vi "App.vi"() -> ()   [LabVIEW 2015]
uses:
  <vilib>/DAQmx/read.llb/DAQmx Read (Analog DBL 1Chan 1Samp).vi
  <vilib>/DAQmx/read.llb/DAQmx Read (Analog Wfm 1Chan NSamp).vi
  <vilib>/DAQmx/miscellaneous.llb/DAQmx Fill In Error Info.vi
panel:
  in  "task out":refnum<k21>
  out "Button 2":u16
  out "Waveform Chart 2":waveform(dbl)
  out "Button":u16
  in  "Tab Control":T1(tab)
  in  "Zoom":bool
  in  "Vol (AI3/AI7)":bool
  out "min value":dbl format="%#.2f"
  out "max value":dbl format="%#.2f"
  out "Delta(ms)":dbl format="%#_5f"
  in  "Zero":bool
  out "Average":dbl format="%#_4g"
  in  "mA/uA":bool
  out "Waveform Graph":waveform(dbl)(graph)
  in  "uA/mA":bool=TRUE
  out "Waveform Graph 2":waveform(dbl)(graph)
  out "Average (uA)":dbl
  in  "PAUSE":bool
  out "Vbat":dbl
  out "Waveform Chart":dbl(graph)
  in  "Number of samples uC Board":i32=10000
  in  "USB DAQ":tag="Dev1"
  in  "Stream":bool
  out "Waveform Chart 3":dbl(graph)
  in  "file List":i32(listbox)
  out "2D Picture":picture
  # "FW Validation - Current Tracking V1.0"
  # "For uC Board: 20kS/s"
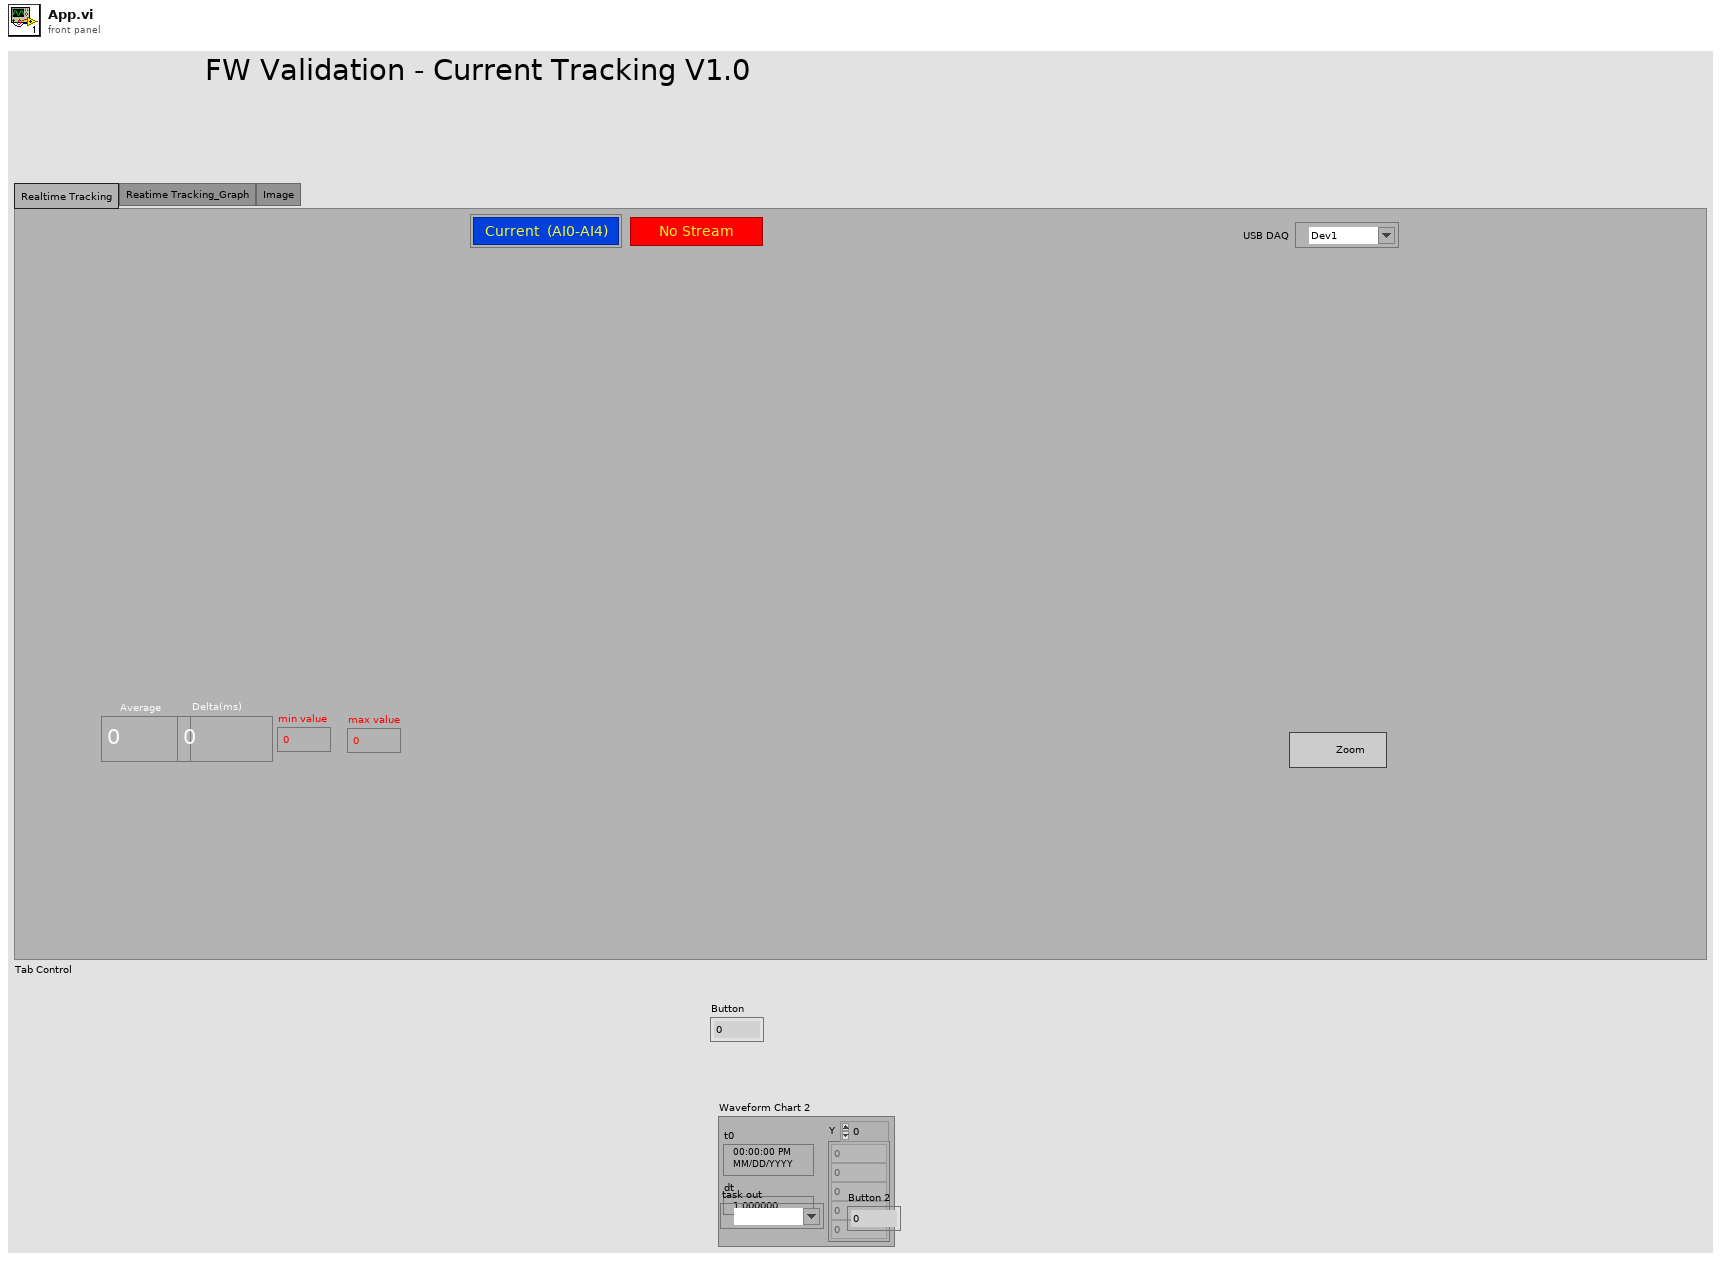
[diagram p1: front panel]
types:
  T1 = enum32{"Realtime Tracking", "Reatime Tracking_Graph", "Image"}
  T2 = typedef "imagedata.ctl" = cluster{"image type":i32, "image depth":i32, "image":u8[], "mask":u8[], "colors":u32[], "Rectangle":cluster{"left":i16, "top":i16, "right":i16, "bottom":i16}}
  T3 = typedef "LVCursorListTypeDef.ctl" = cluster{"Name":string, "Color":u32, "Style":u8, "Point Style":u8, "Name Visible":bool, "Allow Drag":bool, "Cursor Mode":u32, "Plot":i32, "Index":i32, "Position":cluster{"X":dbl, "Y":dbl}, "X Scale":u32, "Y Scale":u32, "Watch Plots":i32[], "Watch All Plots":bool, "Plot Area":i32, "Label Offset":cluster{"X":dbl, "Y":dbl}}[]
  T4 = cluster{"Name":string, "Color":u32, "Style":u8, "Point Style":u8, "Name Visible":bool, "Allow Drag":bool, "Cursor Mode":u32, "Plot":i32, "Index":i32, "Position":cluster{"X":dbl, "Y":dbl}, "X Scale":u32, "Y Scale":u32, "Watch Plots":i32[], "Watch All Plots":bool, "Plot Area":i32, "Label Offset":cluster{"X":dbl, "Y":dbl}}
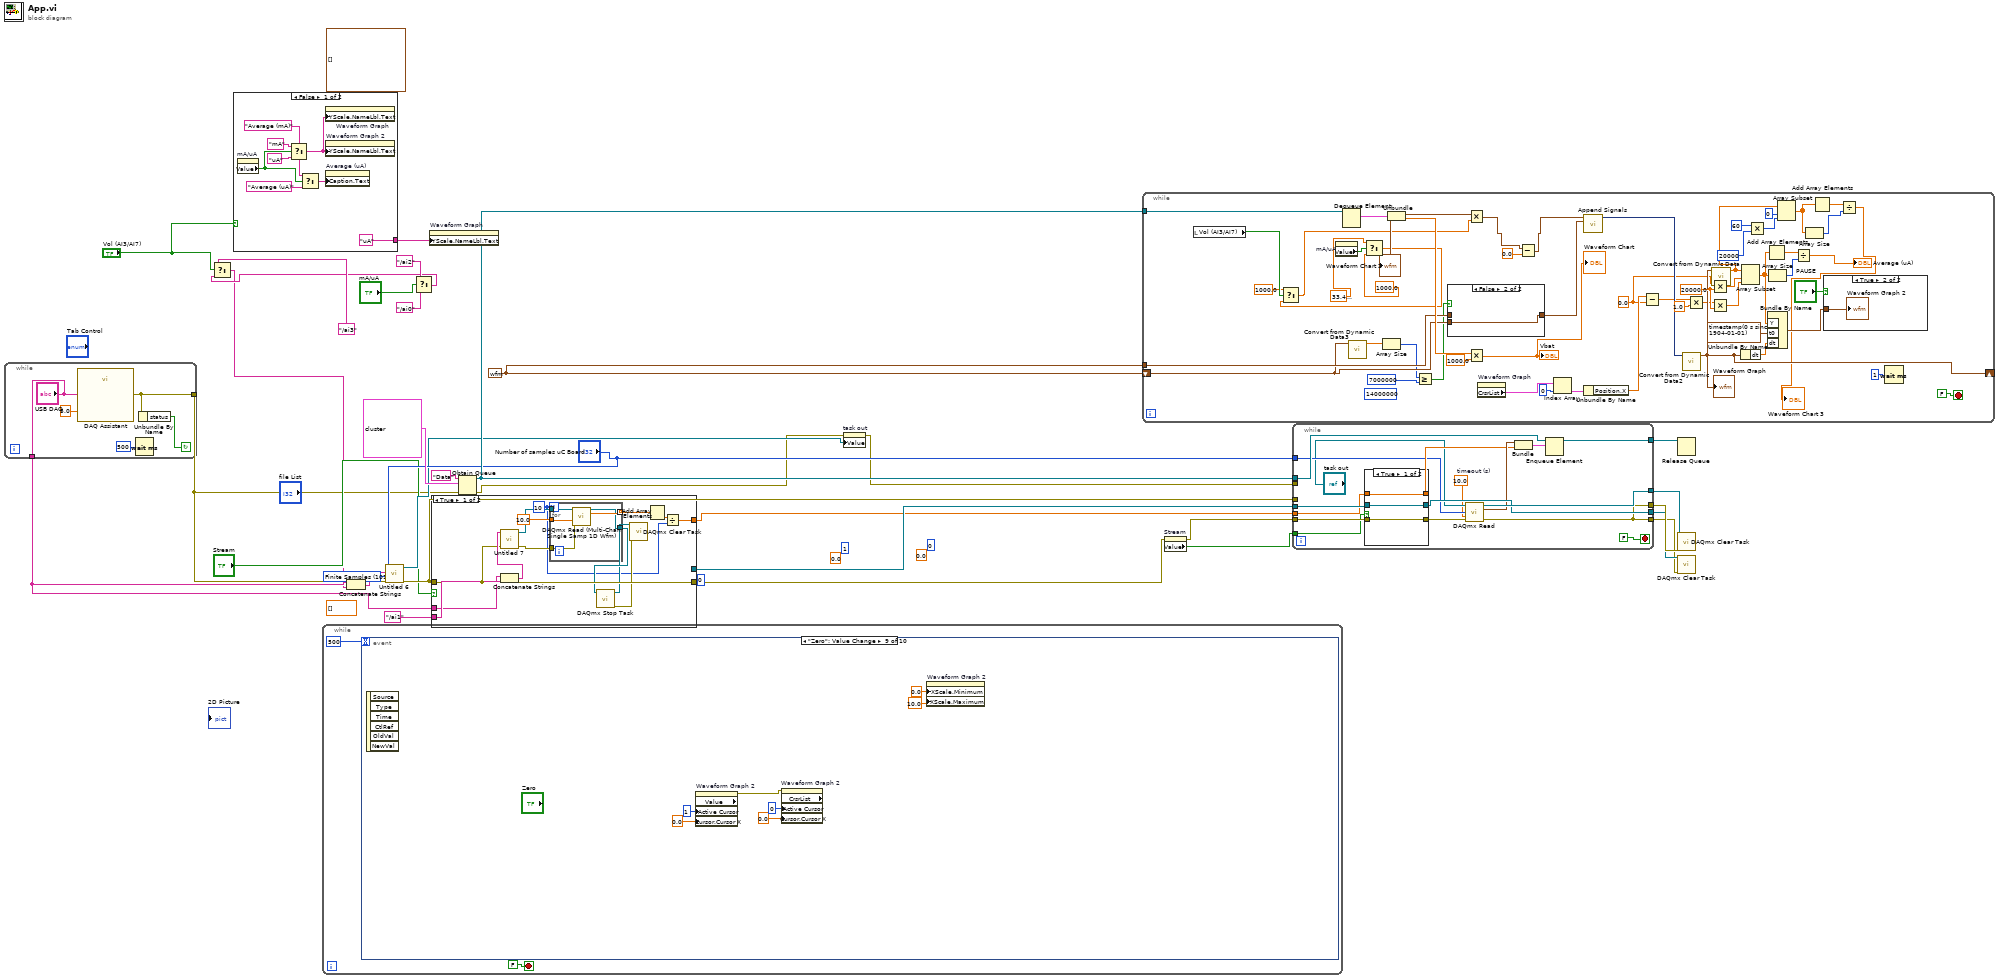
[diagram p0: block diagram]
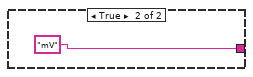
[diagram p2: hidden frame]
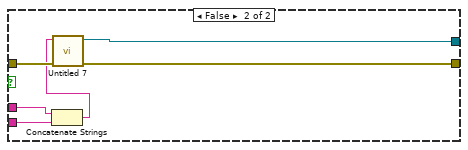
[diagram p3: hidden frame]
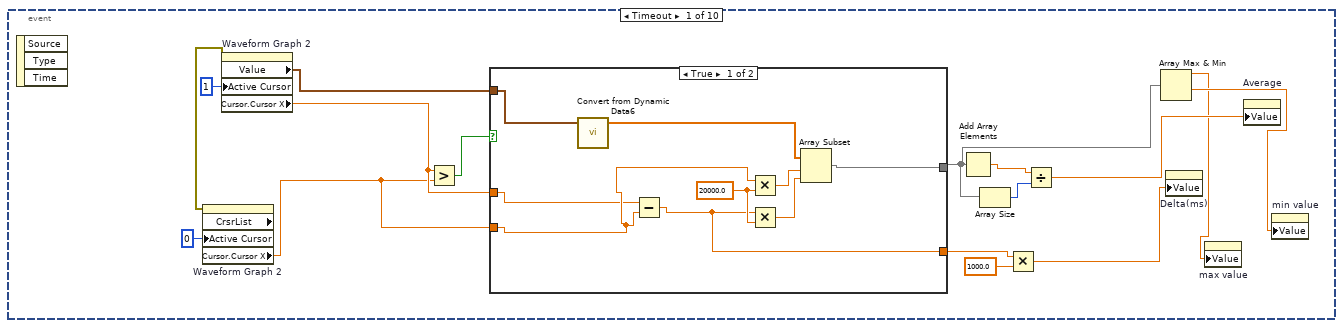
[diagram p4: hidden frame]
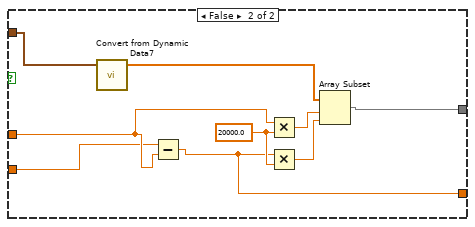
[diagram p5: hidden frame]
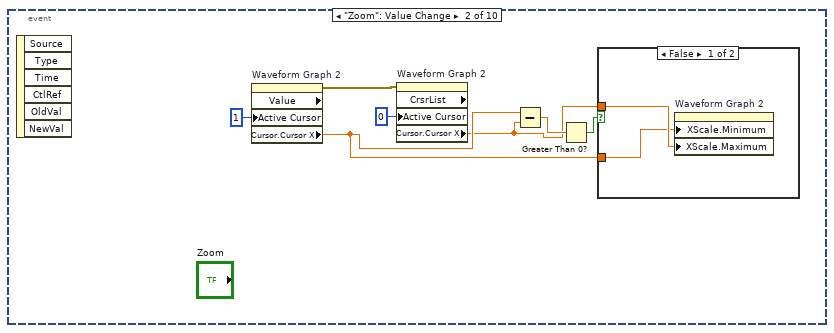
[diagram p6: hidden frame]
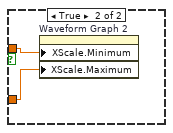
[diagram p7: hidden frame]
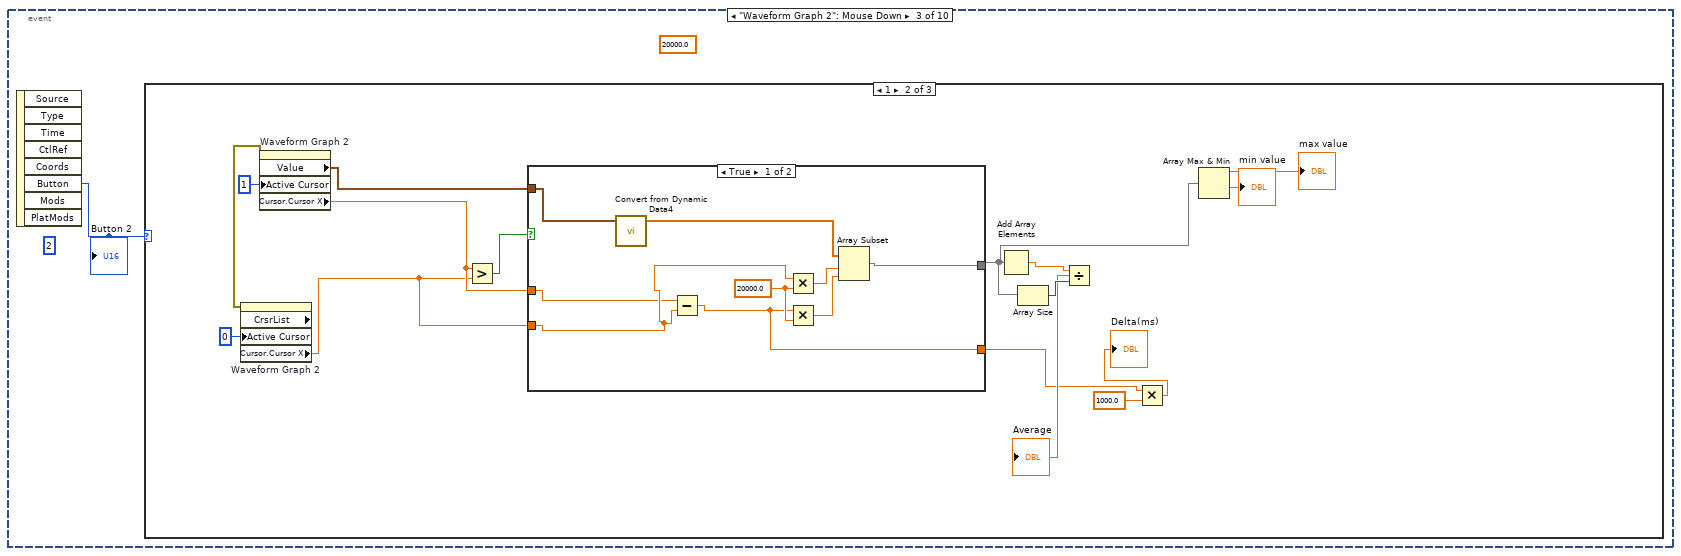
[diagram p8: hidden frame]
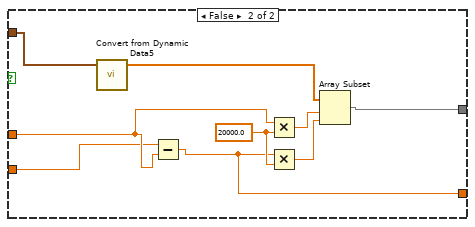
[diagram p10: hidden frame]
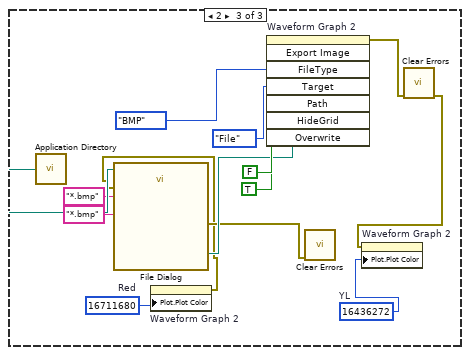
[diagram p11: hidden frame]
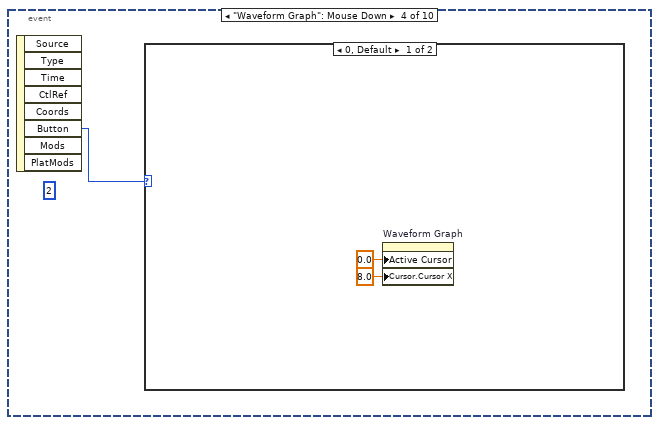
[diagram p12: hidden frame]
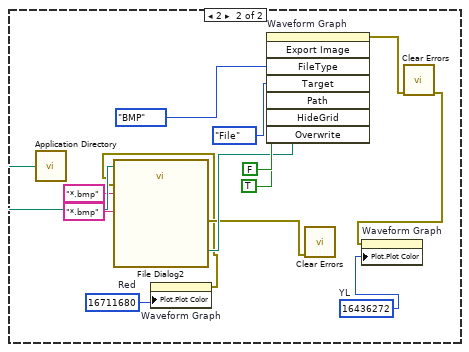
[diagram p13: hidden frame]
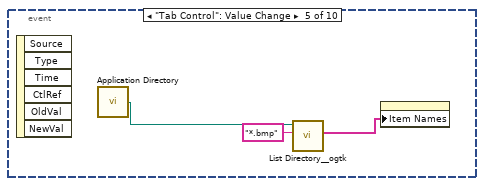
[diagram p14: hidden frame]
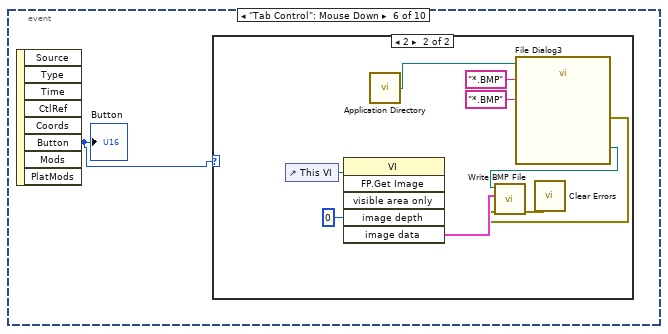
[diagram p15: hidden frame]
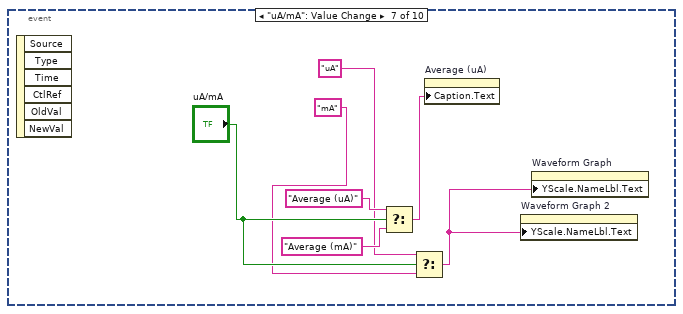
[diagram p17: hidden frame]
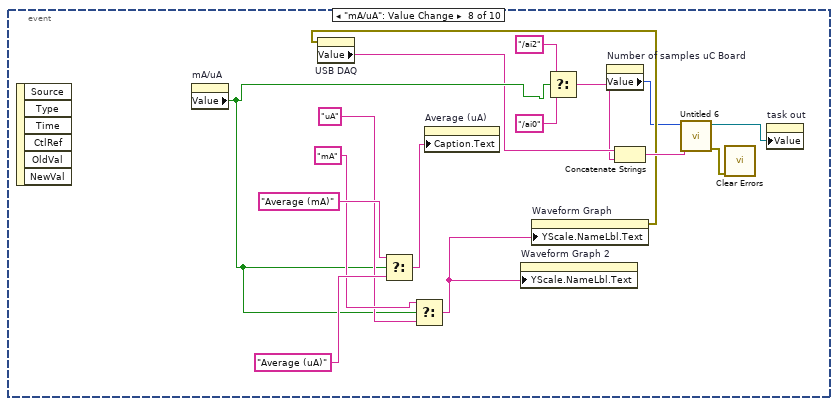
[diagram p18: hidden frame]
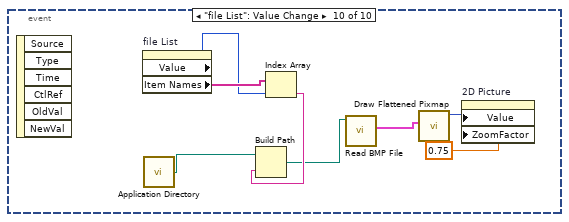
[diagram p19: hidden frame]
diagram:
  (unwired) 0.0 ("Cursor.Cursor Position:Cursor X")
  (unwired) 0.0 ("Cursor.Cursor Position:Cursor X")
  (unwired) u32 0 ("Active Cursor")
  (unwired) u32 1 ("Active Cursor")
  w13 = 10178 items=["Finite Samples"=10178, "Continuous Samples"=10123, "Hardware Timed Single Point"=12522] ("sample mode")
  (unwired) u32 0 ("Active Cursor")
  w23 = waveform(dbl) {"t0"=timestamp(0 s since 1904-01-01), "dt"=0.0, "Y"=[]} ("data")
  (unwired) waveform(dbl)[] [] ("History Data")
  (unwired) dbl[] [] ("Array")
  n1 = while {
    tunnel: [w36] -> w6
    tunnel: ["USB DAQ"] -> w20
    stop <- w35 continue-if-true
    n2 = call "DAQ Assistant"("data"=5.0, "device name"="USB DAQ") -> ("error out"=w36:errorcluster)  [unwired: 16 in, 1 out]
    n3 = Wait (ms)(milliseconds to wait=u32 500) -> ()  [unwired: 1 out]
    n4 = Unbundle By Name(w36) -> ("status"=w35:bool)
  }
  n5 = case shown="False" "Vol (AI3/AI7)" {
    tunnel: ["uA" ("Y Scale.Name Label.Text") "mV" ("Y Scale.Name Label.Text")] -> w1
    frame False {
      n6 = property on="mA/uA" class="Bool (strict)"() -> ("Value"=w43:bool)  [unwired: 2 in, 2 out]
      n7 = Select(t="mA" ("Caption.Text"), s=w43, f="uA" ("Caption.Text")) -> (s? t:f=w44:string)
      n8 = Select(t="Average (mA)" ("Caption.Text"), s=w43, f="Average (uA)" ("Caption.Text")) -> (s? t:f=w45:string)
      n9 = property on="Waveform Graph" class="WFGraph (strict)"("YScale.NameLbl.Text"=w44) -> ()  [unwired: 2 in, 2 out]
      n10 = property on="Waveform Graph 2" class="WFGraph (strict)"("YScale.NameLbl.Text"=w44) -> ()  [unwired: 2 in, 2 out]
      n11 = property on="Average (uA)" class="DigNum (strict)"("Caption.Text"=w45) -> ()  [unwired: 2 in, 2 out]
    }
    frame True {
    }
  }
  n12 = while {
    stop <- FALSE stop-if-true
    n13 = event shown="[8] \"Zero\": Value Change" {
      selector: _ -> [_ _ _ _ _ _ _ _ _ _]
      dyn-events: _ -> [_ _ _ _ _ _ _ _ _ _]
      timeout: 500 -> [_ _ _ _ _ _ _ _ _ _]
      event Timeout {
        n14 = event-data() -> ()  [unwired: 1 in, 3 out]
        n15 = property on="Waveform Graph 2" class="WFGraph (strict)"("Active Cursor"=u32 1) -> (error out=w60:errorcluster, "Value"=w56:waveform(dbl), "Cursor.Cursor X"=w62:dbl)  [unwired: 2 in, 1 out]
        n16 = property on="Waveform Graph 2" class="WFGraph (strict)" props=["CrsrList", "Active Cursor", "Cursor", "Cursor X"](error in=w60, "Active Cursor"=u32 0) -> ("Cursor.Cursor X"=w61:dbl)  [unwired: 1 in, 3 out]
        n17 = Greater?(x=w62, y=w61) -> (0:w63:bool)
        n18 = case shown="True" w63 {
          tunnel: w56 -> [w74 w83]
          tunnel: w62 -> [w67 w77]
          tunnel: w61 -> [w68 w76]
          tunnel: [w69 w78] -> w57
          tunnel: [w66 w75] -> w52
          frame True {
            w72 = 20000.0 ("y")
            n19 = call "Convert from Dynamic Data6"("Dynamic Data Type"=w74) -> ("Array"=w70:dbl[])  [unwired: 3 in]
            n20 = Subtract(x=w67, y=w68) -> (x-y=w66:dbl)
            n21 = Multiply(x=w68, y=w72) -> (x*y=w73:dbl)
            n22 = Multiply(x=w66, y=w72) -> (x*y=w71:dbl)
            n23 = Array Subset(array=w70, index=w73, length=w71) -> (w69:dbl[])
          }
          frame False {
            w81 = 20000.0 ("y")
            n24 = call "Convert from Dynamic Data7"("Dynamic Data Type"=w83) -> ("Array"=w79:dbl[])  [unwired: 3 in]
            n25 = Subtract(x=w76, y=w77) -> (x-y=w75:dbl)
            n26 = Multiply(x=w77, y=w81) -> (x*y=w82:dbl)
            n27 = Multiply(x=w75, y=w81) -> (x*y=w80:dbl)
            n28 = Array Subset(array=w79, index=w82, length=w80) -> (w78:dbl[])
          }
        }
        n29 = Add Array Elements(numeric array=w57) -> (sum=w59:dbl)
        n30 = Array Size(array=w57) -> (size(s)=w58:i32)
        n31 = Multiply(x=w52, y=1000.0) -> (x*y=w51:dbl)
        n32 = Divide(x=w59, y=w58) -> (x/y=w55:dbl)
        n33 = Array Max & Min(array=w57) -> (max value=w53:dbl, min value=w54:dbl)  [unwired: 2 out]
        n34 = property on="Delta(ms)" class="DigNum (strict)"("Value"=w51) -> ()  [unwired: 2 in, 2 out]
        n35 = property on="max value" class="DigNum (strict)"("Value"=w53) -> ()  [unwired: 2 in, 2 out]
        n36 = property on="Average" class="DigNum (strict)"("Value"=w55) -> ()  [unwired: 2 in, 2 out]
        n37 = property on="min value" class="DigNum (strict)"("Value"=w54) -> ()  [unwired: 2 in, 2 out]
      }
      event "Zoom": Value Change {
        n38 = event-data() -> ()  [unwired: 1 in, 6 out]
        n39 = property on="Waveform Graph 2" class="WFGraph (strict)" props=["Value", "Active Cursor", "Cursor", "Cursor X"]("Active Cursor"=u32 1) -> (error out=w88:errorcluster, "Cursor.Cursor X"=w86:dbl)  [unwired: 2 in, 2 out]
        n40 = property on="Waveform Graph 2" class="WFGraph (strict)" props=["CrsrList", "Active Cursor", "Cursor", "Cursor X"](error in=w88, "Active Cursor"=u32 0) -> ("Cursor.Cursor X"=w85:dbl)  [unwired: 1 in, 3 out]
        n41 = Subtract(x=w86, y=w85) -> (x-y=w87:dbl)
        n42 = Greater Than 0?(x=w87) -> (x > 0?=w84:bool)
        n43 = case shown="False" w84 {
          tunnel: w86 -> [w91 w94]
          tunnel: w85 -> [w92 w93]
          frame False {
            n44 = property on="Waveform Graph 2" class="WFGraph (strict)"("XScale.Minimum"=w91, "XScale.Maximum"=w92) -> ()  [unwired: 2 in, 2 out]
          }
          frame True {
            n45 = property on="Waveform Graph 2" class="WFGraph (strict)"("XScale.Minimum"=w93, "XScale.Maximum"=w94) -> ()  [unwired: 2 in, 2 out]
          }
        }
      }
      event "Waveform Graph 2": Mouse Down {
        (unwired) 20000.0 ("y")
        (unwired) u16 2 ("Button")
        n46 = event-data() -> ("Button"=w95:u16)  [unwired: 1 in, 7 out]
        "Button 2" <- w95
        n47 = case shown="1" w95 {
          frame 0, Default {
          }
          frame 1 {
            n48 = property on="Waveform Graph 2" class="WFGraph (strict)"("Active Cursor"=u32 1) -> (error out=w106:errorcluster, "Value"=w99:waveform(dbl), "Cursor.Cursor X"=w108:dbl)  [unwired: 2 in, 1 out]
            n49 = property on="Waveform Graph 2" class="WFGraph (strict)" props=["CrsrList", "Active Cursor", "Cursor", "Cursor X"](error in=w106, "Active Cursor"=u32 0) -> ("Cursor.Cursor X"=w107:dbl)  [unwired: 1 in, 3 out]
            n50 = Greater?(x=w108, y=w107) -> (0:w109:bool)
            n51 = case shown="True" w109 {
              tunnel: w99 -> [w120 w129]
              tunnel: w108 -> [w113 w123]
              tunnel: w107 -> [w114 w122]
              tunnel: [w115 w124] -> w102
              tunnel: [w112 w121] -> w96
              frame True {
                w118 = 20000.0 ("y")
                n52 = call "Convert from Dynamic Data4"("Dynamic Data Type"=w120) -> ("Array"=w116:dbl[])  [unwired: 3 in]
                n53 = Subtract(x=w113, y=w114) -> (x-y=w112:dbl)
                n54 = Multiply(x=w114, y=w118) -> (x*y=w119:dbl)
                n55 = Multiply(x=w112, y=w118) -> (x*y=w117:dbl)
                n56 = Array Subset(array=w116, index=w119, length=w117) -> (w115:dbl[])
              }
              frame False {
                w127 = 20000.0 ("y")
                n57 = call "Convert from Dynamic Data5"("Dynamic Data Type"=w129) -> ("Array"=w125:dbl[])  [unwired: 3 in]
                n58 = Subtract(x=w122, y=w123) -> (x-y=w121:dbl)
                n59 = Multiply(x=w123, y=w127) -> (x*y=w128:dbl)
                n60 = Multiply(x=w121, y=w127) -> (x*y=w126:dbl)
                n61 = Array Subset(array=w125, index=w128, length=w126) -> (w124:dbl[])
              }
            }
            n62 = Add Array Elements(numeric array=w102) -> (sum=w105:dbl)
            n63 = Array Size(array=w102) -> (size(s)=w104:i32)
            n64 = Divide(x=w105, y=w104) -> (x/y=→"Average":dbl)
            n65 = Multiply(x=w96, y=1000.0) -> (x*y=→"Delta(ms)":dbl)
            n66 = Array Max & Min(array=w102) -> (max value=→"max value":dbl, min value=→"min value":dbl)  [unwired: 2 out]
          }
          frame 2 {
            w130 = u32 16436272  # YL
            w132 = u32 16711680  # Red
            n67 = call <vilib>:"Application Directory.vi"() -> ("Application Directory"=w139:path)
            n68 = property on="Waveform Graph 2" class="WFGraph (strict)"("Plot.Plot Color"=w132) -> (error out=w133:errorcluster)  [unwired: 2 in, 1 out]
            n69 = call "File Dialog"("start path"=w139, "error in"=w133, "pattern (all files)"="*.bmp", "pattern label"="*.bmp") -> ("selected path"=w136:path, "error out"=w135:errorcluster)  [unwired: 8 in, 2 out]
            n70 = invoke on="Waveform Graph 2" class="WFGraph (strict)" method="Export Image"("FileType"=enum32{"BMP", "EPS", "EMF", "PICT"}."BMP" ("File Type"), "Target"=enum32{"File", "Clipboard"}."File", "Path"=w136, "HideGrid"=FALSE ("Hide Grid"), "Overwrite"=TRUE ("Always Overwrite")) -> (error out=w134:errorcluster)  [unwired: 3 in, 7 out]
            n71 = call <vilib>:"Clear Errors.vi"("error in (no error)"=w135) -> ()  [unwired: 5 in, 2 out]
            n72 = call <vilib>:"Clear Errors.vi"("error in (no error)"=w134) -> ("error out"=w131:errorcluster)  [unwired: 5 in, 1 out]
            n73 = property on="Waveform Graph 2" class="WFGraph (strict)"(error in=w131, "Plot.Plot Color"=w130) -> ()  [unwired: 1 in, 2 out]
          }
        }
      }
      event "Waveform Graph": Mouse Down {
        (unwired) u16 2 ("Button")
        n74 = event-data() -> ("Button"=w144:u16)  [unwired: 1 in, 7 out]
        n75 = case shown="0, Default" w144 {
          frame 0, Default {
            n76 = property on="Waveform Graph" class="WFGraph (strict)"("Active Cursor"=0.0 ("Cursor.Cursor Position:Cursor X"), "Cursor.Cursor X"=8.0 ("Cursor.Cursor Position:Cursor X")) -> ()  [unwired: 2 in, 2 out]
          }
          frame 2 {
            w147 = u32 16436272  # YL
            w149 = u32 16711680  # Red
            n77 = call <vilib>:"Application Directory.vi"() -> ("Application Directory"=w156:path)
            n78 = property on="Waveform Graph" class="WFGraph (strict)"("Plot.Plot Color"=w149) -> (error out=w150:errorcluster)  [unwired: 2 in, 1 out]
            n79 = call "File Dialog2"("start path"=w156, "error in"=w150, "pattern (all files)"="*.bmp", "pattern label"="*.bmp") -> ("selected path"=w153:path, "error out"=w152:errorcluster)  [unwired: 8 in, 2 out]
            n80 = invoke on="Waveform Graph" class="WFGraph (strict)" method="Export Image"("FileType"=enum32{"BMP", "EPS", "EMF", "PICT"}."BMP" ("File Type"), "Target"=enum32{"File", "Clipboard"}."File", "Path"=w153, "HideGrid"=FALSE ("Hide Grid"), "Overwrite"=TRUE ("Always Overwrite")) -> (error out=w151:errorcluster)  [unwired: 3 in, 7 out]
            n81 = call <vilib>:"Clear Errors.vi"("error in (no error)"=w152) -> ()  [unwired: 5 in, 2 out]
            n82 = call <vilib>:"Clear Errors.vi"("error in (no error)"=w151) -> ("error out"=w148:errorcluster)  [unwired: 5 in, 1 out]
            n83 = property on="Waveform Graph" class="WFGraph (strict)"(error in=w148, "Plot.Plot Color"=w147) -> ()  [unwired: 1 in, 2 out]
          }
        }
      }
      event "Tab Control": Value Change {
        n84 = event-data() -> ()  [unwired: 1 in, 6 out]
        n85 = call <vilib>:"Application Directory.vi"() -> ("Application Directory"=w163:path)
        n86 = call <userlib>:"List Directory__ogtk.vi"("pattern"="*.bmp", "directory path"=w163) -> ("file names"=w161:string[])  [unwired: 2 in, 3 out]
        n87 = property on="file List" class="LstBox (strict)"("Item Names"=w161) -> ()  [unwired: 2 in, 2 out]
      }
      event "Tab Control": Mouse Down {
        n88 = event-data() -> ("Button"=w164:u16)  [unwired: 1 in, 7 out]
        "Button" <- w164
        n89 = case shown="2" w164 {
          frame 0, Default {
          }
          frame 2 {
            n90 = control-ref of="This VI"() -> (w173:refnum<vi>)
            n91 = invoke class="VI" method="FP.Get Image"(reference=w173, "image depth"=0 ("Image Depth")) -> ("image data"=w171:T2)  [unwired: 4 in, 5 out]
            n92 = call <vilib>:"Application Directory.vi"() -> ("Application Directory"=w167:path)
            n93 = call "File Dialog3"("start path"=w167, "pattern (all files)"="*.BMP", "pattern label"="*.BMP") -> ("selected path"=w170:path, "error out"=w169:errorcluster)  [unwired: 9 in, 2 out]
            n94 = call <vilib>:"Write BMP File.vi"("error in (no error)"=w169, "image data"=w171, "path to BMP file"=w170) -> ("error out"=w165:errorcluster)  [unwired: 7 in, 1 out]
            n95 = call <vilib>:"Clear Errors.vi"("error in (no error)"=w165) -> ()  [unwired: 5 in, 2 out]
          }
        }
      }
      event "uA/mA": Value Change {
        n96 = event-data() -> ()  [unwired: 1 in, 6 out]
        n97 = Select(t="Average (uA)" ("Caption.Text"), s="uA/mA", f="Average (mA)" ("Caption.Text")) -> (s? t:f=w180:string)
        n98 = Select(t="uA" ("Caption.Text"), s="uA/mA", f="mA" ("Caption.Text")) -> (s? t:f=w174:string)
        n99 = property on="Average (uA)" class="DigNum (strict)"("Caption.Text"=w180) -> ()  [unwired: 2 in, 2 out]
        n100 = property on="Waveform Graph 2" class="WFGraph (strict)"("YScale.NameLbl.Text"=w174) -> ()  [unwired: 2 in, 2 out]
        n101 = property on="Waveform Graph" class="WFGraph (strict)"("YScale.NameLbl.Text"=w174) -> ()  [unwired: 2 in, 2 out]
      }
      event "mA/uA": Value Change {
        n102 = event-data() -> ()  [unwired: 1 in, 6 out]
        n103 = property on="mA/uA" class="Bool (strict)"() -> ("Value"=w188:bool)  [unwired: 2 in, 2 out]
        n104 = Select(t="Average (mA)" ("Caption.Text"), s=w188, f="Average (uA)" ("Caption.Text")) -> (s? t:f=w196:string)
        n105 = Select(t="mA" ("Caption.Text"), s=w188, f="uA" ("Caption.Text")) -> (s? t:f=w195:string)
        n106 = property on="Average (uA)" class="DigNum (strict)"("Caption.Text"=w196) -> ()  [unwired: 2 in, 2 out]
        n107 = property on="Waveform Graph 2" class="WFGraph (strict)"("YScale.NameLbl.Text"=w195) -> ()  [unwired: 2 in, 2 out]
        n108 = property on="Waveform Graph" class="WFGraph (strict)"("YScale.NameLbl.Text"=w195) -> (error out=w184:errorcluster)  [unwired: 2 in, 1 out]
        n109 = property on="USB DAQ" class="DAQmxName"(error in=w184) -> ("Value"=w186:string)  [unwired: 1 in, 2 out]
        n110 = Select(t="/ai2" ("string"), s=w188, f="/ai0" ("string")) -> (s? t:f=w185:string)
        n111 = property on="Number of samples uC Board" class="DigNum (strict)"() -> ("Value"=w183:i32)  [unwired: 2 in, 2 out]
        n112 = Concatenate Strings(w186, w185) -> (w187:string)
        n113 = call "Untitled 6.vi"("physical channel"=w187, "number of samples"=w183) -> ("error out"=w181:errorcluster, "task out"=w182:refnum<k21>)  [unwired: 8 in]
        n114 = call <vilib>:"Clear Errors.vi"("error in (no error)"=w181) -> ()  [unwired: 5 in, 2 out]
        n115 = property on="task out" class="DAQmxName (strict)"("Value"=w182) -> ()  [unwired: 2 in, 2 out]
      }
      event "Zero": Value Change {
        n116 = event-data() -> ()  [unwired: 1 in, 6 out]
        n117 = property on="Waveform Graph 2" class="WFGraph (strict)" props=["Value", "Active Cursor", "Cursor", "Cursor X"]("Active Cursor"=u32 1, "Cursor.Cursor X"=0.0 ("Cursor.Cursor Position:Cursor X")) -> (error out=w201:errorcluster)  [unwired: 2 in, 2 out]
        n118 = property on="Waveform Graph 2" class="WFGraph (strict)" props=["CrsrList", "Active Cursor", "Cursor", "Cursor X"](error in=w201, "Active Cursor"=u32 0, "Cursor.Cursor X"=0.0 ("Cursor.Cursor Position:Cursor X")) -> ()  [unwired: 1 in, 3 out]
        n119 = property on="Waveform Graph 2" class="WFGraph (strict)"("XScale.Minimum"=0.0 ("X Scale.Range:Minimum"), "XScale.Maximum"=10.0 ("X Scale.Range:Maximum")) -> ()  [unwired: 2 in, 2 out]
      }
      event "file List": Value Change {
        n120 = event-data() -> ()  [unwired: 1 in, 6 out]
        n121 = property on="file List" class="LstBox (strict)"() -> ("Value"=w210:i32, "Item Names"=w211:string[])  [unwired: 2 in, 2 out]
        n122 = call <vilib>:"Application Directory.vi"() -> ("Application Directory"=w207:path)
        n123 = Index Array(array=w211, index=w210) -> (element=w206:string)
        n124 = Build Path(base path=w207, name or relative path=w206) -> (appended path=w205:path)
        n125 = call <vilib>:"Read BMP File.vi"("path to BMP file"=w205) -> ("image data"=w209:T2)  [unwired: 8 in, 2 out]
        n126 = call <vilib>:"Draw Flattened Pixmap.vi"("image data"=w209) -> ("new picture"=w208:picture)  [unwired: 8 in]
        n127 = property on="2D Picture" class="Pict"("Value"=w208, "ZoomFactor"=sgl 0.75 ("Zoom Factor")) -> ()  [unwired: 2 in, 2 out]
      }
    }
  }
  n128 = Select(t="/ai2" ("string"), s="mA/uA", f="/ai0" ("string")) -> (s? t:f=w4:string)
  n129 = Select(t="/ai3" ("string"), s="Vol (AI3/AI7)", f=w4) -> (s? t:f=w3:string)
  n130 = Concatenate Strings(w20, w3) -> (w21:string)
  n131 = call "Untitled 6.vi"("error in"=w6, "sample mode"=w13, "physical channel"=w21, "number of samples"="Number of samples uC Board") -> ("error out"=w25:errorcluster, "task out"=w16:refnum<k21>)  [unwired: 6 in]
  n132 = property on="Waveform Graph" class="WFGraph (strict)"("YScale.NameLbl.Text"=w1) -> ()  [unwired: 2 in, 2 out]
  n133 = case shown="True" "Stream" {
    tunnel: [_ w236] -> w28
    tunnel: [w223 w235] -> w10
    tunnel: w25 -> [w223 w234]
    tunnel: w20 -> [w212 w233]
    tunnel: "/ai1" ("string") -> [w224 w231]
    tunnel: [w213 _] -> w7
    frame True {
      w214 = 10
      n134 = Concatenate Strings(w212, w224) -> (w225:string)
      n135 = call "Untitled 7.vi"("error in"=w223, "physical channel"=w225) -> ("error out"=w220:errorcluster, "task out"=w222:refnum<k21>)  [unwired: 8 in]
      n136 = for {
        N: w214 -> [_]
        tunnel: w222 -> [w230]
        tunnel: 10.0 ("timeout") -> [w229]
        tunnel: w220 -> [w228]
        tunnel: [w227] -> w216 mode=indexing
        tunnel: [w226] -> w219
        n137 = call-poly "DAQmx Read (Multi-Chan Single Samp 1D Wfm).vi"("task/channels in"=w230, "timeout"=w229, "error in"=w228) -> ("task out"=w226:refnum<k21>, "data"=w227:dbl)  [unwired: 10 in, 1 out]
      }
      n138 = call <vilib>:"DAQmx Stop Task.vi"("task/channels in"=w219) -> ("task out"=w218:refnum<k21>, "error out"=w217:errorcluster)  [unwired: 13 in]
      n139 = call <vilib>:"DAQmx Clear Task.vi"("task in"=w218, "error in"=w217) -> ()  [unwired: 13 in, 1 out]
      n140 = Add Array Elements(numeric array=w216) -> (sum=w215:dbl)
      n141 = Divide(x=w215, y=w214) -> (x/y=w213:dbl)
    }
    frame False {
      n142 = Concatenate Strings(w233, w231) -> (w232:string)
      n143 = call "Untitled 7.vi"("error in"=w234, "physical channel"=w232) -> ("error out"=w235:errorcluster, "task out"=w236:refnum<k21>)  [unwired: 8 in]
    }
  }
  n144 = Obtain Queue(name (unnamed)="Data", element data type=cluster{"Waveform Chart 2":waveform(dbl), dbl} {"Waveform Chart 2"={"t0"=timestamp(0 s since 1904-01-01), "dt"=1.0, "Y"=[]}, 0.0}, error in (no error)=w6) -> (queue out=w30:refnum<queue>, error out=w15:errorcluster)  [unwired: 2 in, 1 out]
  n145 = property on="task out" class="DAQmxName (strict)"(error in=w15, "Value"=w16) -> (error out=w14:errorcluster)  [unwired: 1 in, 1 out]
  n146 = while {
    tunnel: w30 -> [w291]
    shift-right: [w280] -> _
    shift-left: w23 -> [w260]
    tunnel: w23 -> [w261]
    stop <- FALSE stop-if-true
    (unwired) 14000000 ("size(s)")
    w270 = 0.0
    w284 = 20000.0 ("y")
    n147 = local read "Vol (AI3/AI7)"() -> (w240:bool)
    n148 = property on="mA/uA" class="Bool (strict)"() -> ("Value"=w252:bool)  [unwired: 2 in, 2 out]
    n149 = Dequeue Element(queue=w291) -> (element=w267:cluster{"Waveform Chart 2":waveform(dbl), dbl})  [unwired: 2 in, 3 out]
    n150 = call "Convert from Dynamic Data3"("Dynamic Data Type"=w260) -> ("Array"=w259:dbl[])  [unwired: 3 in]
    n151 = Select(t=33.499999999999986 ("y"), s=w252, f=1000.0 ("y")) -> (s? t:f=w238:dbl)
    n152 = Select(t=1000.0, s=w240, f=w238) -> (s? t:f=w237:dbl)
    n153 = Array Size(array=w259) -> (size(s)=w258:i32)
    n154 = Unbundle(w267) -> ("Waveform Chart 2"=w266:waveform(dbl), w265:dbl)
    "Waveform Chart 2" <- w266
    n155 = Greater Or Equal?(x=w258, y=7000000 ("size(s)")) -> (x >= y?=w256:bool)
    n156 = case shown="False" w256 {
      tunnel: w260 -> [_ w293]
      tunnel: [w292 w293] -> w262
      tunnel: w261 -> [w292 _]
      frame True {
      }
      frame False {
      }
    }
    n157 = Multiply(x=w266, y=w237) -> (x*y=w253:waveform(dbl))
    n158 = Multiply(x=w265, y=1000.0) -> (x*y=→"Vbat" →"Waveform Chart":dbl)
    n159 = property on="Waveform Graph" class="WFGraph (strict)"() -> ("CrsrList"=w287:T3)  [unwired: 2 in, 2 out]
    n160 = Subtract(x=w253, y=0.0) -> (x-y=w254:waveform(dbl))
    n161 = Index Array(array=w287, index=0) -> (element=w268:T4)
    n162 = call "Append Signals"("Input Signal B"=w262, "Input Signal A"=w254) -> ("Appended Signals"=w288:dynamicdata)  [unwired: 8 in, 1 out]
    n163 = Unbundle By Name(w268) -> ("Position.X"=w271:dbl)
    n164 = Subtract(x=w271, y=w270) -> (x-y=w274:dbl)
    n165 = call "Convert from Dynamic Data2"("Dynamic Data Type"=w288) -> ("Waveform"=w280:waveform(dbl))  [unwired: 3 in]
    "Waveform Graph" <- w280
    n166 = Multiply(x=w274, y=1.0) -> (x*y=w272:dbl)
    n167 = Multiply(x=w270, y=w284) -> (x*y=w285:dbl)
    n168 = Multiply(x=w272, y=w284) -> (x*y=w283:dbl)
    n169 = call "Convert from Dynamic Data"("Dynamic Data Type"=w280) -> ("Array"=w248:dbl[])  [unwired: 3 in]
    n170 = Unbundle By Name(w280) -> ("dt"=w279:dbl)
    n171 = Array Subset(array=w248, index=w285, length=w283) -> (w278:dbl[])
    n172 = Multiply(x=60, y=20000) -> (x*y=w244:i32)
    n173 = Add Array Elements(numeric array=w278) -> (sum=w277:dbl)
    n174 = Bundle By Name("Y"=w278, "t0"=timestamp(0 s since 1904-01-01), "dt"=w279) -> (w282:waveform(dbl))  [unwired: 1 in]
    n175 = Array Size(array=w278) -> (size(s)=w276:i32)
    n176 = Array Subset(array=w248, index=0, length=w244) -> (w247:dbl[])
    n177 = Divide(x=w277, y=w276) -> (x/y=→"Average (uA)":dbl)
    n178 = Array Size(array=w247) -> (size(s)=w246:i32)
    n179 = Add Array Elements(numeric array=w247) -> (sum=w249:dbl)
    n180 = case shown="True" "PAUSE" {
      tunnel: w282 -> [_ w294]
      frame False {
      }
      frame True {
        "Waveform Graph 2" <- w294
      }
    }
    n181 = Divide(x=w249, y=w246) -> (x/y=→"Waveform Chart 3":dbl)
    n182 = Wait (ms)(milliseconds to wait=u32 1) -> ()  [unwired: 1 out]
  }
  n183 = property on="Stream" class="Bool (strict)"(error in=w10) -> (error out=w9:errorcluster, "Value"=w8:bool)  [unwired: 1 in, 1 out]
  n184 = while {
    tunnel: w25 -> [_]
    tunnel: [w311] -> w33
    tunnel: [w303] -> w32
    tunnel: w30 -> [w310]
    tunnel: [w309] -> w29
    tunnel: w28 -> [w307]
    tunnel: w9 -> [w306]
    tunnel: [w305] -> w27
    tunnel: [w303] -> w26
    tunnel: "Number of samples uC Board" -> [w299]
    tunnel: w14 -> [_]
    tunnel: w8 -> [w297]
    tunnel: w7 -> [w296]
    stop <- FALSE ("stop (F)") stop-if-true
    w295 = 10.0  # timeout (s)
    n185 = case shown="True" w297 {
      tunnel: w307 -> [w313 w319]
      tunnel: w306 -> [w312 w318]
      tunnel: [w313 w317] -> w305
      tunnel: [w312 w316] -> w304
      tunnel: [w314 w315] -> w301
      tunnel: w296 -> [w314 _]
      frame True {
      }
      frame False {
        n186 = call-poly "DAQmx Read (Multi-Chan Single Samp 1D Wfm).vi"("task/channels in"=w319, "error in"=w318) -> ("task out"=w317:refnum<k21>, "data"=w315:dbl, "error out"=w316:errorcluster)  [unwired: 11 in]
      }
    }
    n187 = call-poly <vilib>:"DAQmx Read.vi"("task/channels in"="task out", "number of samples per channel"=w299, "timeout"=w295, "error in"=w304) -> ("task out"=w311:refnum<k21>, "data"=w302:waveform(dbl), "error out"=w303:errorcluster)  [unwired: 9 in]
    n188 = Bundle("data"=w302, "data"=w301) -> (w300:cluster{"data":waveform(dbl), "data":dbl})  [unwired: 1 in]
    n189 = Enqueue Element(queue=w310, element=w300) -> (queue out=w309:refnum<queue>)  [unwired: 2 in, 2 out]
  }
  n190 = Release Queue(queue=w29) -> ()  [unwired: 2 in, 3 out]
  n191 = call <vilib>:"DAQmx Clear Task.vi"("task in"=w33, "error in"=w32) -> ()  [unwired: 13 in, 1 out]
  n192 = call <vilib>:"DAQmx Clear Task.vi"("task in"=w27, "error in"=w26) -> ()  [unwired: 13 in, 1 out]
